vi "circular_shooter_angle_calc.vi"(0 "Current Position":dbl, 1 "Driver Input":dbl, 2 "Upper Bound":dbl, 3 "Lower Bound":dbl, 4 "Scale Factor":dbl, 5 "dt":dbl, 6 "Reset":bool, 7 "P":dbl, 8 "Max Velocity":dbl, 9 "I":dbl, 10 "Low Angle":bool, 11 "D":dbl, 12 "High Angle":bool) -> (14 "Motor Voltage Out":dbl)   [LabVIEW 2012]
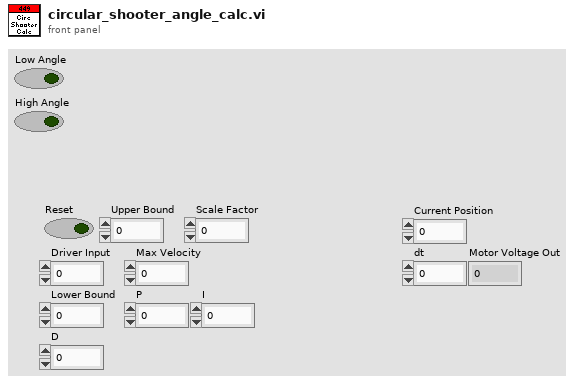
[diagram p1: front panel]
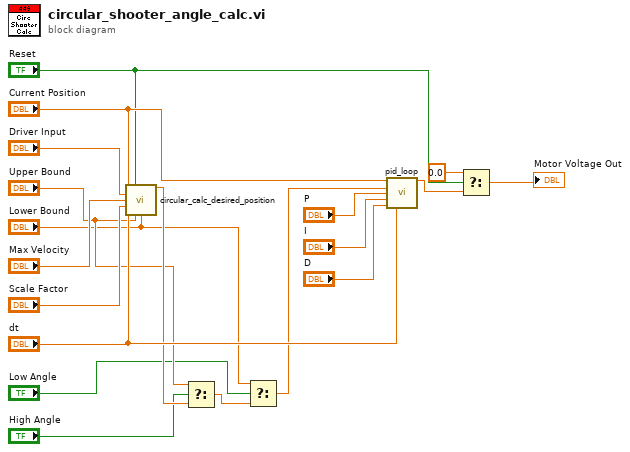
[diagram p0: block diagram]
diagram:
  n1 = call "circular_calc_desired_position.vi"("Current Position"="Current Position", "Reset"="Reset", "Driver Input"="Driver Input", "Max Velocity"="Max Velocity", "Scale Factor"="Scale Factor", "dt"="dt", "Upper Bound"="Upper Bound", "Lower Bound"="Lower Bound") -> ("Desired Position"=w7:dbl)  [unwired: 7 in]
  n2 = Select(t="Upper Bound", s="High Angle", f=w7) -> (s? t:f=w4:dbl)
  n3 = Select(t="Lower Bound", s="Low Angle", f=w4) -> (s? t:f=w1:dbl)
  n4 = call "pid_loop.vi"("Current Pos"="Current Position", "Desired Pos"=w1, "P"="P", "I"="I", "D"="D", "dt"="dt") -> ("Voltage Output"=w11:dbl)  [unwired: 9 in]
  n5 = Select(t=0.0, s="Reset", f=w11) -> (s? t:f=→"Motor Voltage Out":dbl)
